vi "ProgressBar engine.vi"(8 "error in (no error)":errorcluster, 11 "ProgressBar in":refnum<class "ProgressBar.lvclass">) -> (0 "error out":errorcluster, 3 "ProgressBar out":refnum<class "ProgressBar.lvclass">)   [LabVIEW 2018, in "ProgressBar.lvclass"]
uses:
  ProgressBar.lvclass
  ProgressBar.lvclass/ProgressBar.ctl
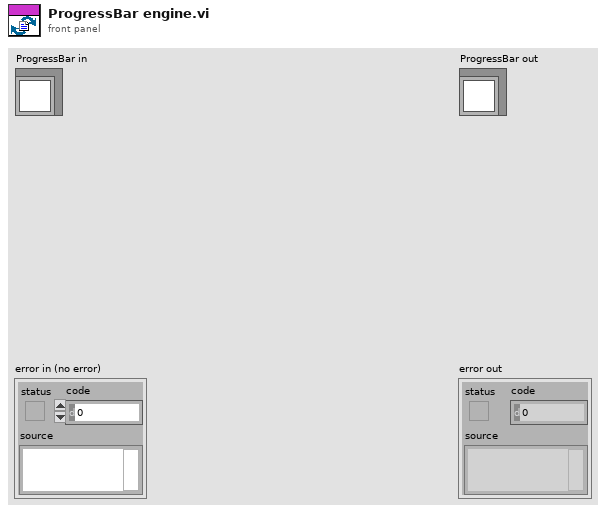
[diagram p1: front panel]
types:
  T1 = enum8{"Enabled", "Disabled", "Disabled and Grayed Out"}
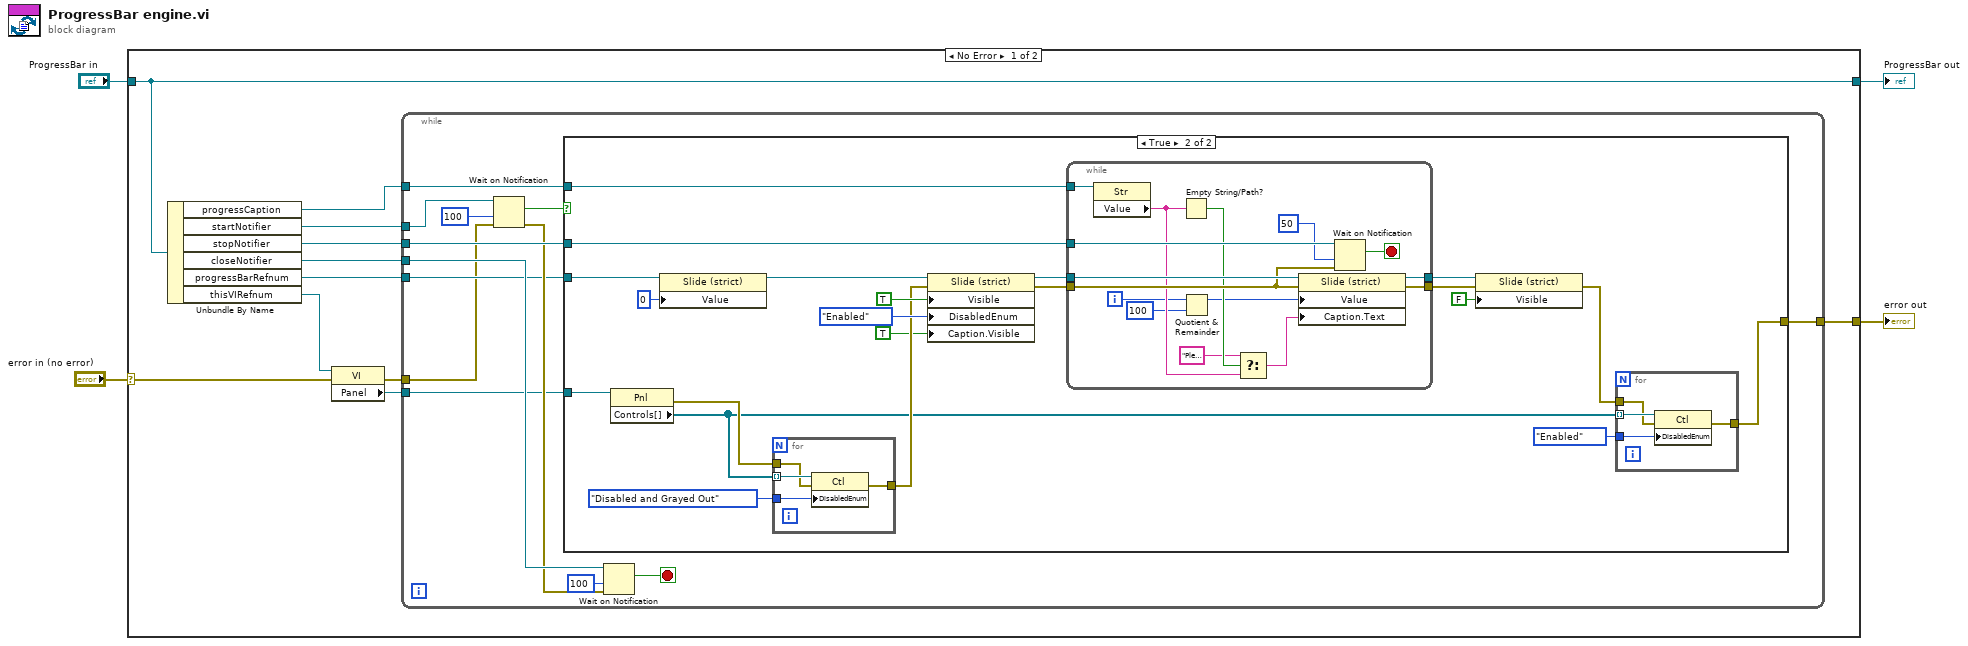
[diagram p0: block diagram]
diagram:
  n1 = case shown="No Error" "error in (no error)" {
    selector: "error in (no error)" -> [w7 w74]
    tunnel: [w6 w74] -> w3
    tunnel: [w15 w73] -> w1
    tunnel: "ProgressBar in" -> [w15 w73]
    frame No Error {
      n2 = Unbundle By Name(w15) -> ("progressCaption"=w5:refnum<vi>, "startNotifier"=w14:refnum<notifier>, "stopNotifier"=w13:refnum<notifier>, "closeNotifier"=w12:refnum<notifier>, "progressBarRefnum"=w9:refnum<vi>, "thisVIRefnum"=w11:refnum<vi>)
      n3 = property class="VI"(reference=w11, error in=w7) -> (error out=w8:errorcluster, "Panel"=w10:refnum<vi>)  [unwired: 1 out]
      n4 = while {
        tunnel: w14 -> [w28]
        tunnel: w13 -> [w22]
        tunnel: w12 -> [w27]
        tunnel: w10 -> [w20]
        tunnel: w9 -> [w19]
        tunnel: w8 -> [w18]
        tunnel: [w17] -> w6
        tunnel: w5 -> [w16]
        stop <- w26 stop-if-true
        n5 = Wait on Notification(notifier=w28, timeout in ms (-1)=100, error in (no error)=w18) -> (notification=w23:bool, error out=w21:errorcluster)  [unwired: 1 in, 2 out]
        n6 = case shown="True" w23 {
          tunnel: w22 -> [_ w46]
          tunnel: w20 -> [_ w49]
          tunnel: w19 -> [_ w43]
          tunnel: [_ w32] -> w17
          tunnel: w16 -> [_ w30]
          frame False {
          }
          frame True {
            n7 = property class="Pnl"(reference=w49) -> (error out=w47:errorcluster, "Controls[]"=w34:refnum<vi>[])  [unwired: 1 in, 1 out]
            n8 = property class="Slide (strict)"(reference=w43, "Value"=0) -> (reference out=w41:refnum<vi>)  [unwired: 1 in, 1 out]
            n9 = for {
              tunnel: w34 -> [w72] mode=indexing
              tunnel: T1."Disabled and Grayed Out" ("Disabled") -> [w71]
              tunnel: [w70] -> w40
              tunnel: w47 -> [w69]
              n10 = property class="Ctl"(reference=w72, error in=w69, "DisabledEnum"=w71) -> (error out=w70:errorcluster)  [unwired: 1 out]
            }
            n11 = property class="Slide (strict)"(reference=w41, error in=w40, "Visible"=TRUE, "DisabledEnum"=T1."Enabled" ("Disabled"), "Caption.Visible"=TRUE) -> (reference out=w39:refnum<vi>, error out=w38:errorcluster)
            n12 = while {
              tunnel: w46 -> [w68]
              tunnel: w39 -> [w65]
              tunnel: [w64] -> w36
              tunnel: [w63] -> w35
              tunnel: w38 -> [w62]
              tunnel: w30 -> [w61]
              i -> [w56]
              stop <- w67 stop-if-true
              n13 = property class="Str"(reference=w61) -> ("Value"=w59:string)  [unwired: 1 in, 2 out]
              n14 = Empty String/Path?(string/path=w59) -> (empty?=w60:bool)
              n15 = Quotient & Remainder(x=w56, y=100) -> (x-y*floor(x/y)=w54:i32)  [unwired: 1 out]
              n16 = Select(t="Please Wait...", s=w60, f=w59) -> (s? t:f=w57:string)
              n17 = property class="Slide (strict)"(reference=w65, error in=w62, "Value"=w54, "Caption.Text"=w57) -> (reference out=w64:refnum<vi>, error out=w63:errorcluster)
              n18 = Wait on Notification(notifier=w68, timeout in ms (-1)=50, error in (no error)=w62) -> (notification=w67:bool)  [unwired: 1 in, 3 out]
            }
            n19 = property class="Slide (strict)"(reference=w36, error in=w35, "Visible"=FALSE) -> (error out=w31:errorcluster)  [unwired: 1 out]
            n20 = for {
              tunnel: w34 -> [w53] mode=indexing
              tunnel: T1."Enabled" ("Disabled") -> [w52]
              tunnel: w31 -> [w51]
              tunnel: [w50] -> w32
              n21 = property class="Ctl"(reference=w53, error in=w51, "DisabledEnum"=w52) -> (error out=w50:errorcluster)  [unwired: 1 out]
            }
          }
        }
        n22 = Wait on Notification(notifier=w27, timeout in ms (-1)=100, error in (no error)=w21) -> (notification=w26:bool)  [unwired: 1 in, 3 out]
      }
    }
    frame Error {
    }
  }
  "error out" <- w3
  "ProgressBar out" <- w1
